vi "Motor speed test.vi"() -> ()   [LabVIEW 2015]
uses:
  Robot Values.vi
  <vilib>/ptbypt/NI_PtbyPt.lvlib
panel:
  in  "PbP 2":enum16{"Mean", "Median", "None"}(ring)
  in  "sample length 2":i32=25
  out "x/y 2":dbl
  out "x-y 2":dbl
  out "x/y":dbl
  in  "PbP":enum16{"Mean", "Median", "None"}(ring)
  in  "sample length":i32=25
  out "x-y":dbl
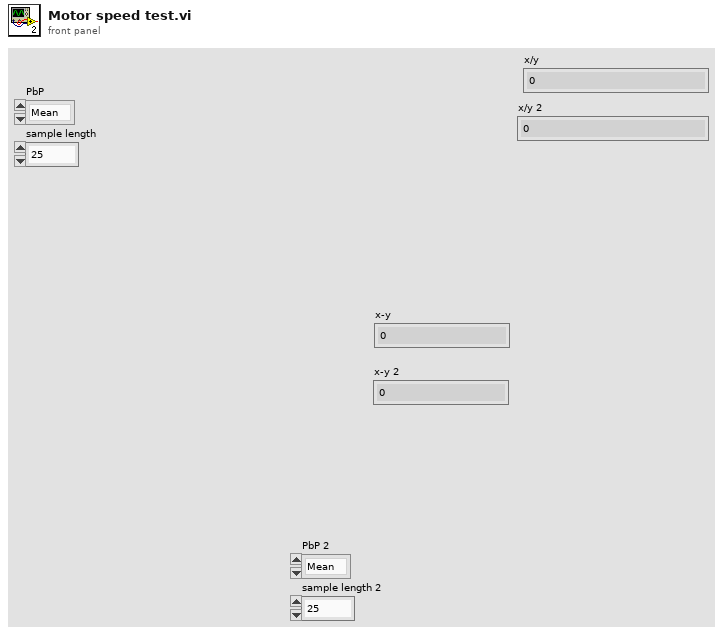
[diagram p1: front panel]
types:
  T1 = typedef "Robot Values.ctl" = cluster{"Drive Motors":cluster{"Left Motor Value":dbl, "Right Motor Value":dbl, "Left Motor Encoder":dbl, "Right Motor Encoder":dbl, "High/Low Gear":bool}, "Sensors":cluster{"Gyro Angle":dbl, "Photoeye":bool, "Ultrasonic Range":dbl, "Shooter Speed Encoder":dbl, "Accelerometer Value":dbl, "Flashlight":bool}, "Arms":cluster{"Desired Arm Position":dbl, "Left Arm Encoder":dbl, "Right Arm Encoder":dbl, "Left Arm Lower Limit":bool, "Right Arm Lower Limit":bool}, "Acquisition and Scoring":cluster{"Acquiring?":bool, "Current Speed":dbl, "Setpoint Speed":dbl, "Prep Wheels":bool, "Shoot":bool, "Low Eject":bool}, "Hanging":cluster{"Pivot Arms":dbl, "PTO":bool, "Left Pivot Encoder":dbl, "Right Pivot Encoder":dbl, "Hanging Pin":bool}}
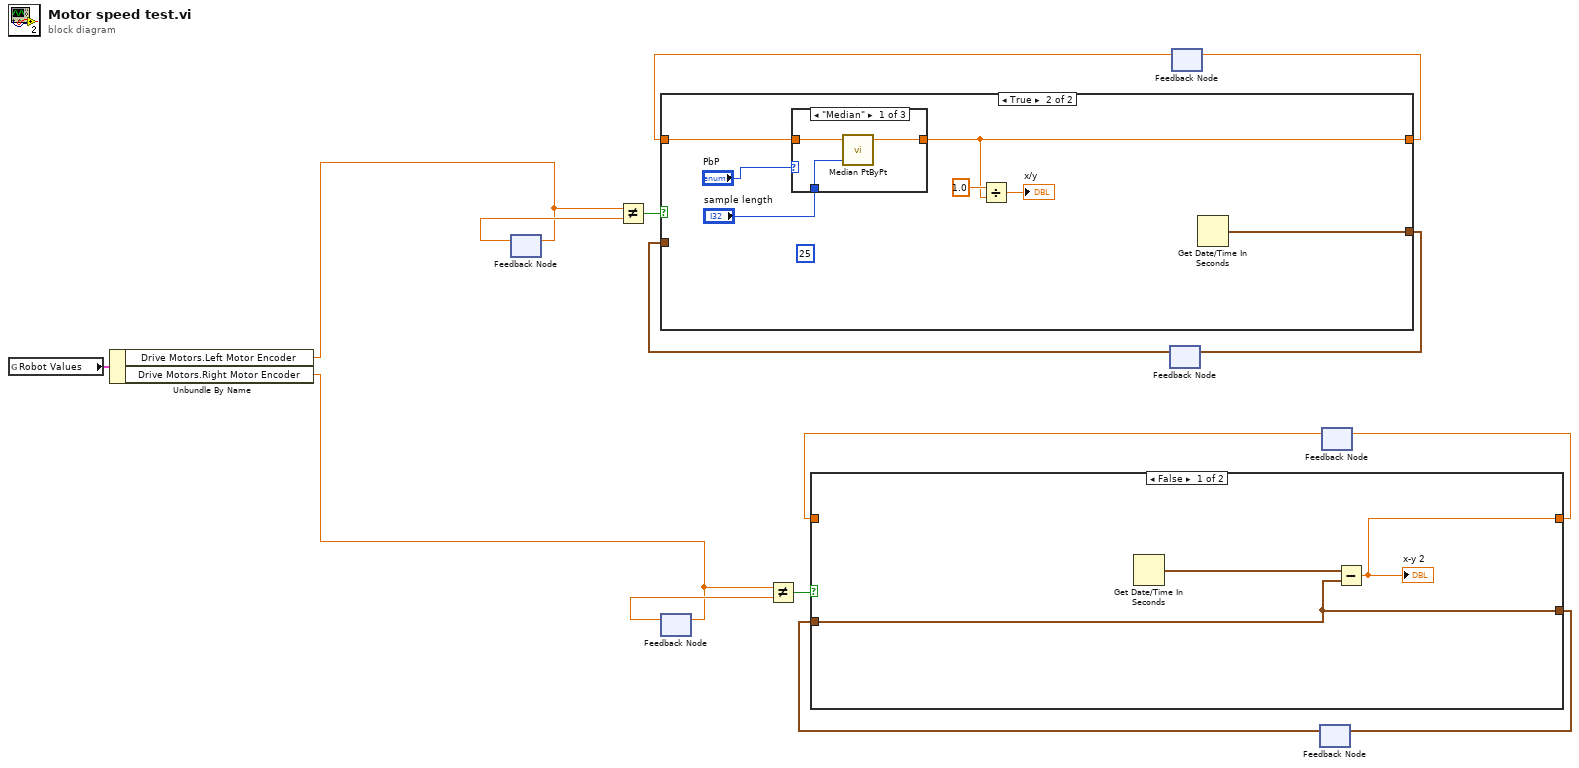
[diagram p0: block diagram]
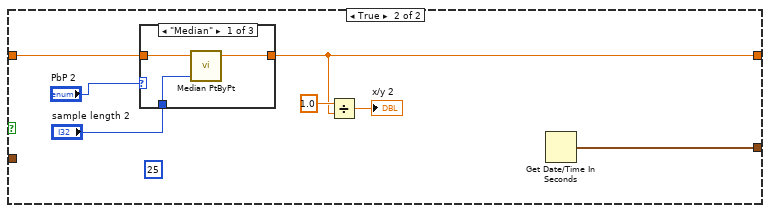
[diagram p2: hidden frame]
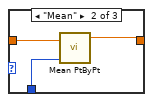
[diagram p3: hidden frame]
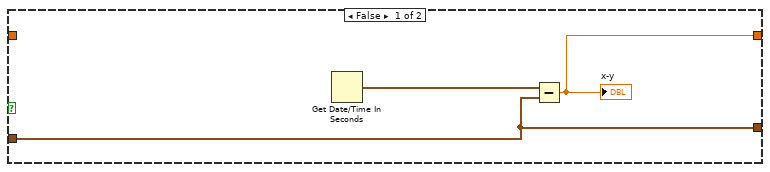
[diagram p5: hidden frame]
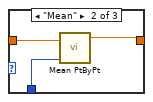
[diagram p6: hidden frame]
diagram:
  n1 = global read "Robot Values.vi" "Robot Values"() -> (w9:T1)
  n2 = Unbundle By Name(w9) -> ("Drive Motors.Left Motor Encoder"=w8:dbl, "Drive Motors.Right Motor Encoder"=w1:dbl)
  n3 = feedback #1() -> (w11:dbl)  [unwired: 1 in]
  n4 = feedback-in #1(w8) -> ()
  n5 = Not Equal?(x=w8, y=w11) -> (x != y?=w12:bool)
  n6 = feedback #2() -> (w3:dbl)  [unwired: 1 in]
  n7 = feedback-in #2(w1) -> ()
  n8 = Not Equal?(x=w1, y=w3) -> (x != y?=w4:bool)
  n9 = feedback #3() -> (w14:timestamp)  [unwired: 1 in]
  n10 = feedback #4() -> (w13:dbl)  [unwired: 1 in]
  n11 = case shown="True" w12 {
    tunnel: [w17 w25] -> w15
    tunnel: w14 -> [w17 _]
    tunnel: [w16 w22] -> w10
    tunnel: w13 -> [_ w23]
    frame False {
      n12 = Get Date/Time In Seconds() -> (seconds since 1Jan1904=w18:timestamp)
      n13 = Subtract(x=w18, y=w17) -> (x-y=w16:dbl)
      "x-y" <- w16
    }
    frame True {
      (unwired) 25 ("sample length")
      n14 = case shown="\"Median\"" "PbP" {
        tunnel: w23 -> [w28 w31 w32]
        tunnel: [w27 w30 w32] -> w22
        tunnel: "sample length" -> [w26 w29 _]
        frame "Median" {
          n15 = call <vilib>:"Median PtByPt.vi"("sample length"=w26, "x"=w28) -> ("median"=w27:dbl)  [unwired: 2 in, 1 out]
        }
        frame "Mean" {
          n16 = call <vilib>:"Mean PtByPt.vi"("x"=w31, "sample length"=w29) -> ("mean"=w30:dbl)  [unwired: 2 in, 1 out]
        }
        frame "None" {
        }
      }
      n17 = Divide(x=1.0, y=w22) -> (x/y=→"x/y":dbl)
      n18 = Get Date/Time In Seconds() -> (seconds since 1Jan1904=w25:timestamp)
    }
  }
  n19 = feedback-in #3(w15) -> ()
  n20 = feedback-in #4(w10) -> ()
  n21 = feedback #5() -> (w6:timestamp)  [unwired: 1 in]
  n22 = feedback #6() -> (w5:dbl)  [unwired: 1 in]
  n23 = case shown="False" w4 {
    tunnel: [w34 w42] -> w7
    tunnel: w6 -> [w34 _]
    tunnel: [w33 w39] -> w2
    tunnel: w5 -> [_ w40]
    frame False {
      n24 = Get Date/Time In Seconds() -> (seconds since 1Jan1904=w35:timestamp)
      n25 = Subtract(x=w35, y=w34) -> (x-y=w33:dbl)
      "x-y 2" <- w33
    }
    frame True {
      (unwired) 25 ("sample length")
      n26 = case shown="\"Median\"" "PbP 2" {
        tunnel: w40 -> [w45 w48 w49]
        tunnel: [w44 w47 w49] -> w39
        tunnel: "sample length 2" -> [w43 w46 _]
        frame "Median" {
          n27 = call <vilib>:"Median PtByPt.vi"("sample length"=w43, "x"=w45) -> ("median"=w44:dbl)  [unwired: 2 in, 1 out]
        }
        frame "Mean" {
          n28 = call <vilib>:"Mean PtByPt.vi"("x"=w48, "sample length"=w46) -> ("mean"=w47:dbl)  [unwired: 2 in, 1 out]
        }
        frame "None" {
        }
      }
      n29 = Divide(x=1.0, y=w39) -> (x/y=→"x/y 2":dbl)
      n30 = Get Date/Time In Seconds() -> (seconds since 1Jan1904=w42:timestamp)
    }
  }
  n31 = feedback-in #5(w7) -> ()
  n32 = feedback-in #6(w2) -> ()
